vi "make burst envelope array.vi"(0 "delay (ms)":dbl format="%.2f", 1 "burst type":T1(ring), 2 "actual sample rate (Hz)":dbl=20000.0 format="%.1f", 3 "samples":i32=16384, 5 "on duration (ms)":dbl format="%.2f", 7 "on + off duration (ms)":dbl format="%.2f", 9 "rise/fall time (ms)":dbl format="%.2f", 11 "number of bursts":dbl format="%.2f", 12 "polarity":enum16{"positive", "negative", "alternate"}(ring)=enum."alternate", 13 "sync to stimulus":enum16{"unlocked", "locked"}(ring)) -> (4 "burst array out":dbl[](array[numeric]) format="%.2f")   [LabVIEW 2015]
uses:
  <vilib>/Analysis/1siggen.llb/Ramp Pattern by Samples.vi
  <vilib>/Analysis/NI_AALBase.lvlib
panel:
  out "# points out":i32
  out "Waveform Plot":cluster{i32, dbl, dbl[]}(graph)
  out "Burst Envelope Array in points":dbl[](graph)
  # "BURSTING"
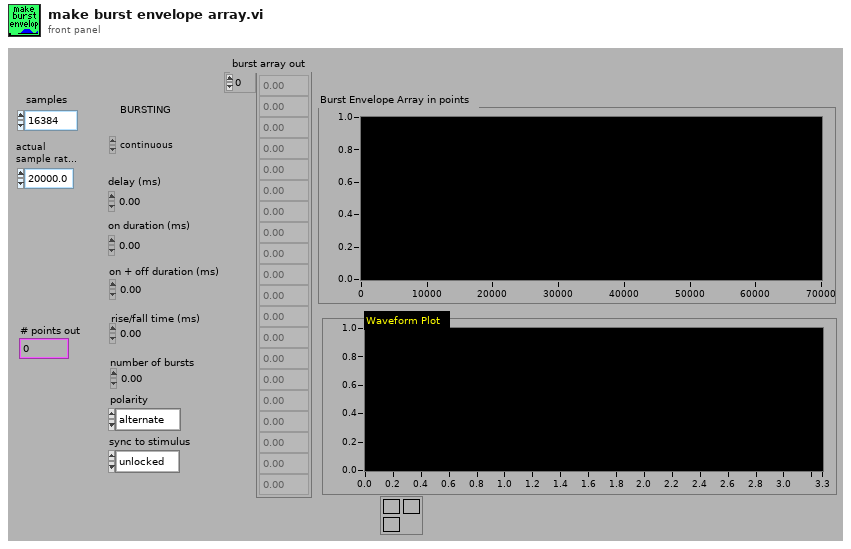
[diagram p1: front panel]
types:
  T1 = enum16{"continuous", "linear ramp", "cosine ramp", "rectangular"}
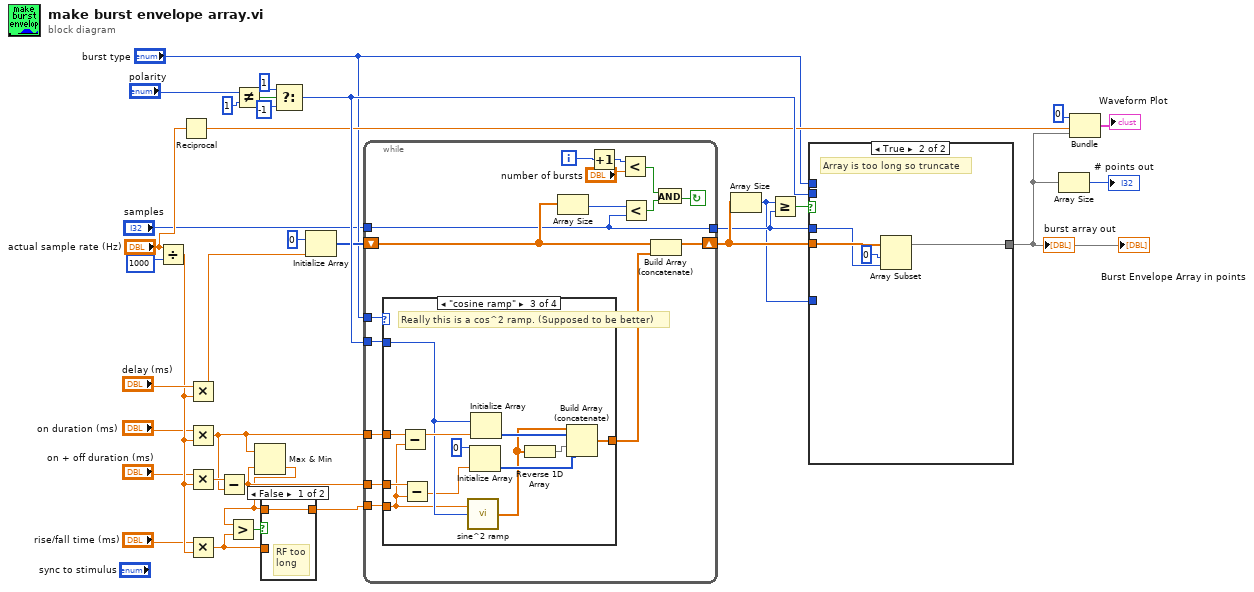
[diagram p0: block diagram]
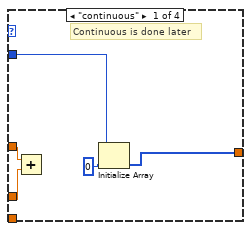
[diagram p2: hidden frame]
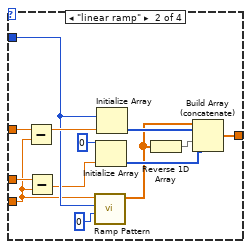
[diagram p3: hidden frame]
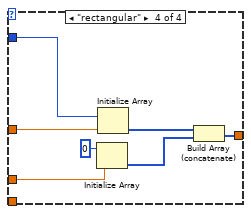
[diagram p4: hidden frame]
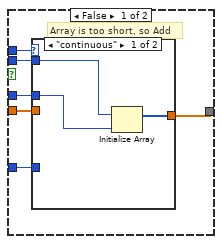
[diagram p6: hidden frame]
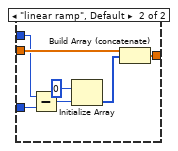
[diagram p7: hidden frame]
diagram:
  n1 = Divide(x="actual sample rate (Hz)", y=1000) -> (x/y=w28:dbl)
  n2 = Reciprocal(x="actual sample rate (Hz)") -> (1/x=w17:dbl)
  n3 = Multiply(x="delay (ms)", y=w28) -> (x*y=w26:dbl)
  n4 = Multiply(x="on duration (ms)", y=w28) -> (x*y=w6:dbl)
  n5 = Multiply(x="on + off duration (ms)", y=w28) -> (x*y=w25:dbl)
  n6 = Multiply(x="rise/fall time (ms)", y=w28) -> (x*y=w3:dbl)
  n7 = Subtract(x=w25, y=w6) -> (x-y=w9:dbl)
  n8 = Not Equal?(x="polarity", y=1) -> (x != y?=w22:bool)
  n9 = Max & Min(x=w6, y=w9) -> (min(x,y)=w4:dbl)  [unwired: 1 out]
  n10 = Greater?(x=w4, y=w3) -> (0:w5:bool)
  n11 = case shown="False" w5 {
    tunnel: w4 -> [w35 _]
    tunnel: [w35 w36] -> w10
    tunnel: w3 -> [_ w36]
    frame False {
      # "RF too\nlong"
    }
    frame True {
      # "OK"
    }
  }
  n12 = Select(t=1, s=w22, f=-1) -> (s? t:f=w32:i32)
  n13 = Initialize Array(0, w26) -> (w21:i32[])
  n14 = while {
    tunnel: [w39] -> w13
    tunnel: "samples" -> [w39]
    shift-left: w21 -> [w45]
    shift-right: [w47] -> w15
    tunnel: "burst type" -> [w48]
    tunnel: w10 -> [w49]
    tunnel: w9 -> [w50]
    tunnel: w6 -> [w51]
    tunnel: w32 -> [w52]
    i -> [w37]
    stop <- w41 continue-if-true
    n15 = case shown="\"cosine ramp\"" w48 {
      tunnel: w49 -> [_ w59 w72 _]
      tunnel: w52 -> [w57 w63 w75 w85]
      tunnel: w51 -> [w56 w65 w77 w84]
      tunnel: w50 -> [w55 w60 w73 w87]
      tunnel: [w54 w66 w76 w86] -> w46
      frame "continuous" {
        # "Continuous is done later"
        n16 = Add(x=w56, y=w55) -> ()  [unwired: 1 out]
        n17 = Initialize Array(w57, 0) -> (w54:i32[])
      }
      frame "linear ramp" {
        n18 = Subtract(x=w65, y=w59) -> (x-y=w64:dbl)
        n19 = Subtract(x=w60, y=w59) -> (x-y=w58:dbl)
        n20 = call-poly <vilib>:"Ramp Pattern.vi"("start"=0, "end"=w63, "samples"=w59) -> ("Ramp Pattern"=w61:dbl[])  [unwired: 7 in, 1 out]
        n21 = Initialize Array(0, w58) -> (w67:i32[])
        n22 = Initialize Array(w63, w64) -> (w70:i32[])
        n23 = Reverse 1D Array(array=w61) -> (reversed array=w69:dbl[])
        n24 = Build Array (concatenate)(w61, w70, w69, w67) -> (w66:dbl[])
      }
      frame "cosine ramp" {
        # "Really this is a cos^2 ramp. (Supposed to be better)"
        n25 = Subtract(x=w77, y=w72) -> (x-y=w78:dbl)
        n26 = Subtract(x=w73, y=w72) -> (x-y=w71:dbl)
        n27 = call "sine^2 ramp.vi"("End Amp."=w75, "samples"=w72) -> ("sine^2 Ramp"=w74:dbl[])  [unwired: 1 in, 2 out]
        n28 = Initialize Array(0, w71) -> (w79:i32[])
        n29 = Initialize Array(w75, w78) -> (w82:i32[])
        n30 = Reverse 1D Array(array=w74) -> (reversed array=w81:dbl[])
        n31 = Build Array (concatenate)(w74, w82, w81, w79) -> (w76:dbl[])
      }
      frame "rectangular" {
        n32 = Initialize Array(0, w87) -> (w88:i32[])
        n33 = Initialize Array(w85, w84) -> (w83:i32[])
        n34 = Build Array (concatenate)(w83, w88) -> (w86:i32[])
      }
    }
    n35 = Array Size(array=w45) -> (size(s)=w43:i32)
    n36 = Increment(x=w37) -> (x+1=w38:i32)
    n37 = Less?(x=w38, y="number of bursts") -> (x < y?=w40:bool)
    n38 = Less?(x=w43, y=w39) -> (x < y?=w42:bool)
    n39 = Build Array (concatenate)(w45, w46) -> (w47:dbl[])
    n40 = And(x=w40, y=w42) -> (x .and. y?=w41:bool)
  }
  n41 = Array Size(array=w15) -> (size(s)=w2:i32)
  n42 = Greater Or Equal?(x=w2, y=w13) -> (x >= y?=w16:bool)
  n43 = case shown="True" w16 {
    tunnel: w15 -> [w94 w109]
    tunnel: w2 -> [w95 _]
    tunnel: [w93 w108] -> w12
    tunnel: "burst type" -> [w92 _]
    tunnel: w32 -> [w91 _]
    tunnel: w13 -> [w90 w107]
    frame False {
      # "Array is too short, so Add"
      n44 = case shown="\"continuous\"" w92 {
        tunnel: w95 -> [_ w100]
        tunnel: w94 -> [_ w103]
        tunnel: [w97 w101] -> w93
        tunnel: w91 -> [w98 _]
        tunnel: w90 -> [w96 w99]
        frame "continuous" {
          n45 = Initialize Array(w98, w96) -> (w97:i32[])
        }
        frame "linear ramp", Default {
          n46 = Subtract(x=w99, y=w100) -> (x-y=w105:i32)
          n47 = Initialize Array(0, w105) -> (w102:i32[])
          n48 = Build Array (concatenate)(w103, w102) -> (w101:dbl[])
        }
      }
    }
    frame True {
      # "Array is too long so truncate"
      n49 = Array Subset(array=w109, index=0, length=w107) -> (w108:dbl[])
    }
  }
  "burst array out" <- w12
  "Burst Envelope Array in points" <- w12
  n50 = Array Size(array=w12) -> (size(s)=→"# points out":i32)
  n51 = Bundle(0, w17, w12) -> (→"Waveform Plot":cluster{i32, dbl, dbl[]})  [unwired: 1 in]
